vi "Translate Schedule to Teams.vi"(0 "Match Array (indices)":i32[][](array[numeric]), 5 "Team Info Out":T1) -> (4 "Display Headers":string[](array[string])=["Match", "Red", "Blue", "Yellow", "Green"], 6 "String Schedule for Display":string[][](array[string]), 8 "String Schedule":string[][](array[string]), 10 "Team Number Schedule":i32[][](array[numeric]), 15 "RAW Schedule":string[][](array[string]))   [LabVIEW 2013]
uses:
  Team Data Array2.ctl
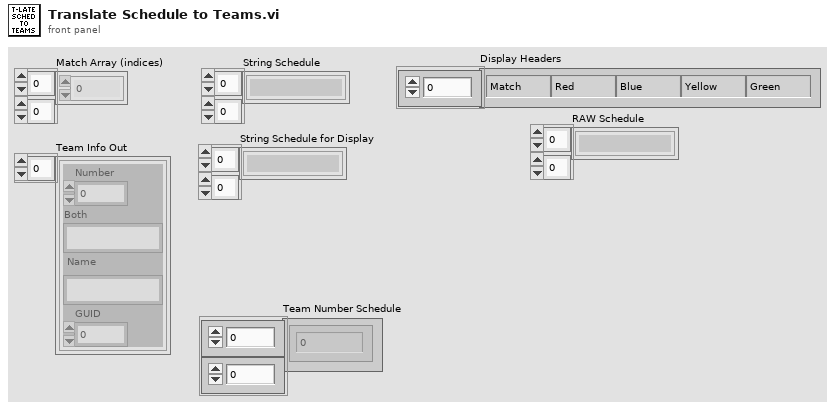
[diagram p1: front panel]
types:
  T1 = typedef "Team Data Array2.ctl" = cluster{"Number":u16, "Both":string, "Name":string, "GUID":u16}[]
  T2 = cluster{"Number":u16, "Both":string, "Name":string, "GUID":u16}
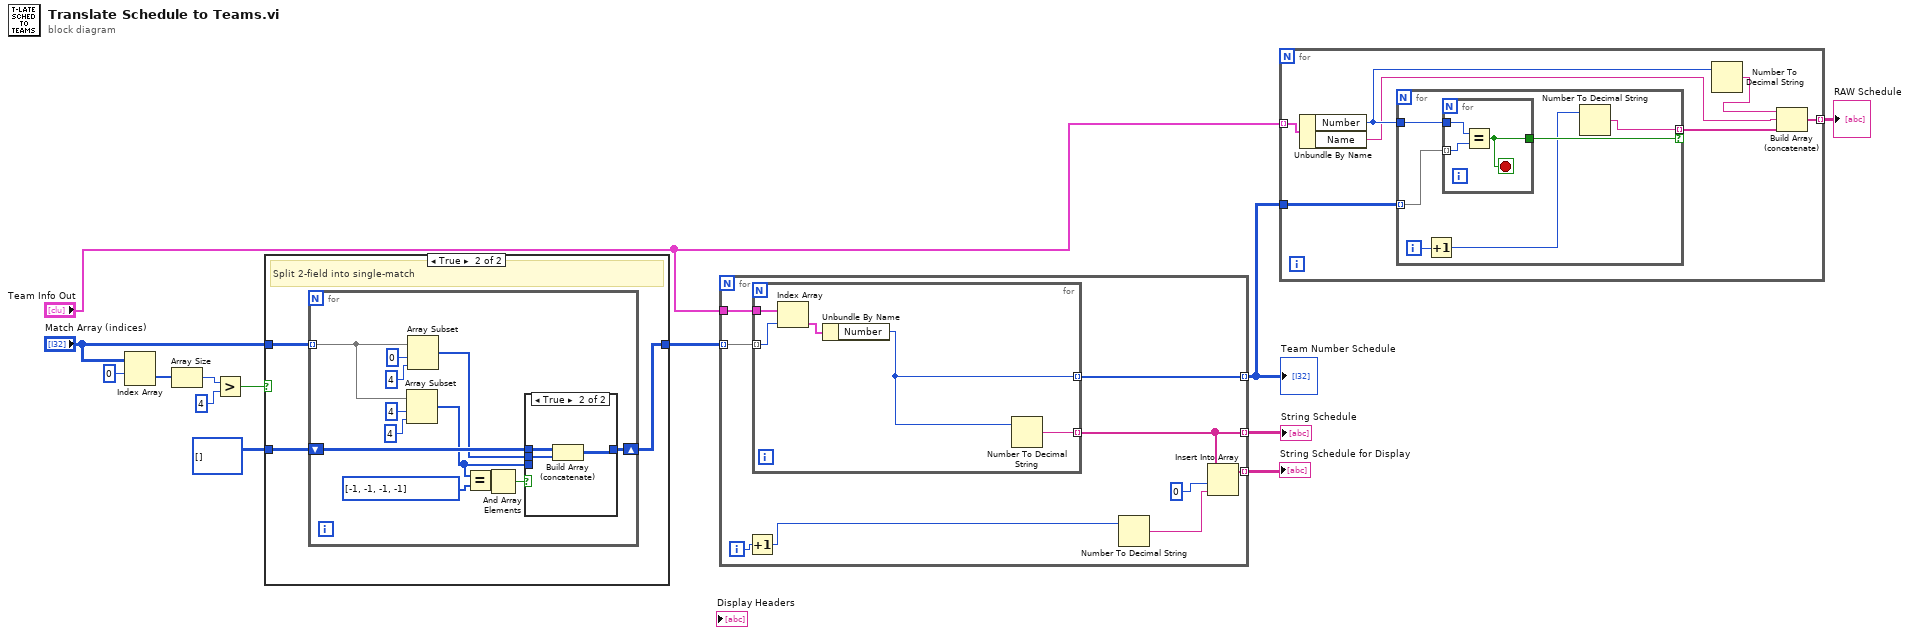
[diagram p0: block diagram]
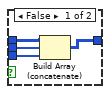
[diagram p3: hidden frame]
diagram:
  n1 = Index Array(array="Match Array (indices)", index (row)=0) -> (element=w10:i32[])  [unwired: 1 in]
  n2 = Array Size(array=w10) -> (size(s)=w9:i32)
  n3 = Greater?(x=w9, y=4) -> (0:w7:bool)
  n4 = case shown="True" w7 {
    tunnel: "Match Array (indices)" -> [w14 w17]
    tunnel: [w14 w15] -> w5
    tunnel: i32[][] [] ("Match Array (indices)") -> [_ w16]
    frame False {
    }
    frame True {
      # "Split 2-field into single-match"
      n5 = for {
        tunnel: w17 -> [w23] mode=indexing
        shift-right: [w22] -> w15
        shift-left: w16 -> [w25]
        n6 = Array Subset(array=w23, index=4, length=4) -> (w20:i32[])
        n7 = Array Subset(array=w23, index=0, length=4) -> (w24:i32[])
        n8 = Equal?(x=w20, y=i32[] [-1, -1, -1, -1]) -> (x = y?=w18:bool[])
        n9 = And Array Elements(Boolean array=w18) -> (logical AND=w19:bool)
        n10 = case shown="True" w19 {
          tunnel: w25 -> [w33 w36]
          tunnel: w24 -> [w32 w35]
          tunnel: w20 -> [w31 _]
          tunnel: [w30 w34] -> w22
          frame False {
            n11 = Build Array (concatenate)(w33, w32, w31) -> (w30:i32[][])
          }
          frame True {
            n12 = Build Array (concatenate)(w36, w35) -> (w34:i32[][])
          }
        }
      }
    }
  }
  n13 = for {
    tunnel: w5 -> [w43] mode=indexing
    tunnel: "Team Info Out" -> [w42]
    tunnel: [w41] -> w13 mode=indexing
    tunnel: [w39] -> w12 mode=indexing
    tunnel: [w38] -> w3 mode=indexing
    i -> [w45]
    n14 = Increment(x=w45) -> (x+1=w44:i32)
    n15 = for {
      tunnel: w43 -> [w50] mode=indexing
      tunnel: w42 -> [w46]
      tunnel: [w48] -> w38 mode=indexing
      tunnel: [w47] -> w41 mode=indexing
      n16 = Index Array(array=w46, index=w50) -> (element=w49:T2)
      n17 = Unbundle By Name(w49) -> ("Number"=w48:u16)
      n18 = Number To Decimal String(number=w48) -> (decimal integer string=w47:string)  [unwired: 1 in]
    }
    n19 = Number To Decimal String(number=w44) -> (decimal integer string=w37:string)  [unwired: 1 in]
    n20 = Insert Into Array(array=w41, index=0, new element=w37) -> (w39:string[])
  }
  "String Schedule" <- w13
  "String Schedule for Display" <- w12
  "Team Number Schedule" <- w3
  n21 = for {
    tunnel: w3 -> [w57]
    tunnel: "Team Info Out" -> [w56] mode=indexing
    tunnel: [w51] -> w1 mode=indexing
    n22 = Unbundle By Name(w56) -> ("Number"=w53:u16, "Name"=w52:string)
    n23 = for {
      tunnel: w57 -> [w63] mode=indexing
      tunnel: w53 -> [w62]
      tunnel: [w60] -> w55 mode=indexing if=w61
      i -> [w59]
      n24 = Increment(x=w59) -> (x+1=w58:i32)
      n25 = for {
        tunnel: w63 -> [w66] mode=indexing
        tunnel: w62 -> [w65]
        tunnel: [w64] -> w61
        stop <- w64 stop-if-true
        n26 = Equal?(x=w65, y=w66) -> (x = y?=w64:bool)
      }
      n27 = Number To Decimal String(number=w58) -> (decimal integer string=w60:string)  [unwired: 1 in]
    }
    n28 = Number To Decimal String(number=w53) -> (decimal integer string=w54:string)  [unwired: 1 in]
    n29 = Build Array (concatenate)(w54, w52, w55) -> (w51:string[])
  }
  "RAW Schedule" <- w1
